vi "test unicode.vi"() -> ()   [LabVIEW 2019]
uses:
  <vilib>/addons/_JKI.lib/Unicode/UTF-8 String/UTF-8 String.lvclass
panel:
  in  "String to be encoded":string="MQIsdp"
  out "error out":errorcluster
  in  "error in (no error)":errorcluster
  out "UTF8 Byte Array":u8[](array[numeric]) format="%x"
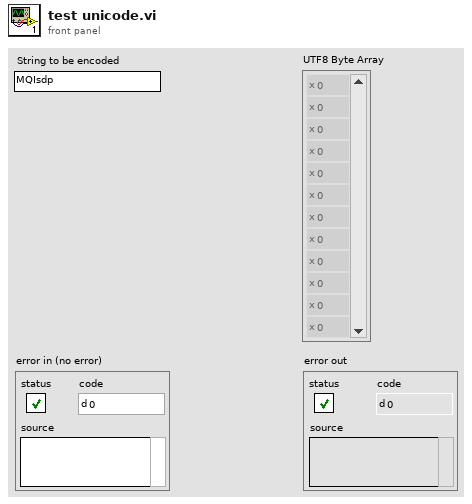
[diagram p1: front panel]
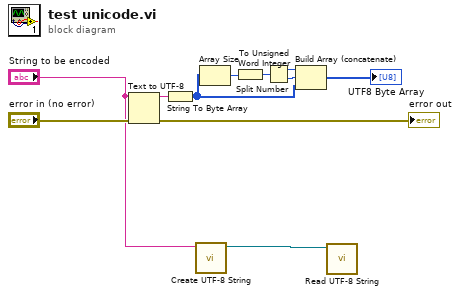
[diagram p0: block diagram]
diagram:
  n1 = Text to UTF-8(8:"error in (no error)", 11:"String to be encoded") -> (0:→"error out":errorcluster, 3:w10:string)  [unwired: 1 in]
  n2 = String To Byte Array(string=w10) -> (unsigned byte array=w9:u8[])
  n3 = call <vilib>:"Create UTF-8 String.vi"("UTF-8 String"="String to be encoded") -> ("UTF-8 String"=w2:refnum<class "UTF-8 String.lvclass">)  [unwired: 9 in, 1 out]
  n4 = Array Size(array=w9) -> (size(s)=w8:i32)
  n5 = To Unsigned Word Integer(number=w8) -> (unsigned 16bit integer=w4:u16)
  n6 = Split Number(x=w4) -> (hi(x)=w6:u8, lo(x)=w7:u8)
  n7 = Build Array (concatenate)(w6, w7, w9) -> (→"UTF8 Byte Array":u8[])
  n8 = call-dynamic "Read UTF-8 String.vi"("UTF8 in"=w2) -> ()  [unwired: 8 in, 3 out]
